vi "GET_OperatorsTable.vi"(8 "error in (no error)":errorcluster, 11 "Database Ref In":T1) -> (0 "error out":errorcluster, 2 "Array":string[][](array[string]), 3 "Database Ref Out":T1)   [LabVIEW 2018, in "MySQLTools.lvlib"]
uses:
  MySQLTools.lvlib
  <vilib>/addons/database/Connection.llb/Conn ObjectReference.ctl
  TypeDefs/DatabaseState.ctl
  <vilib>/addons/database/Recordset.llb/Rec ObjectReference.ctl
  <vilib>/addons/database/Auxilliary.llb/DB Tools Cursor Type.ctl
  <vilib>/addons/database/Connection.llb/Conn Execute.vi
  <vilib>/addons/database/Recordset.llb/Rec Fetch Recordset Data (R).vi
  <vilib>/addons/database/NI_Database_API.lvlib
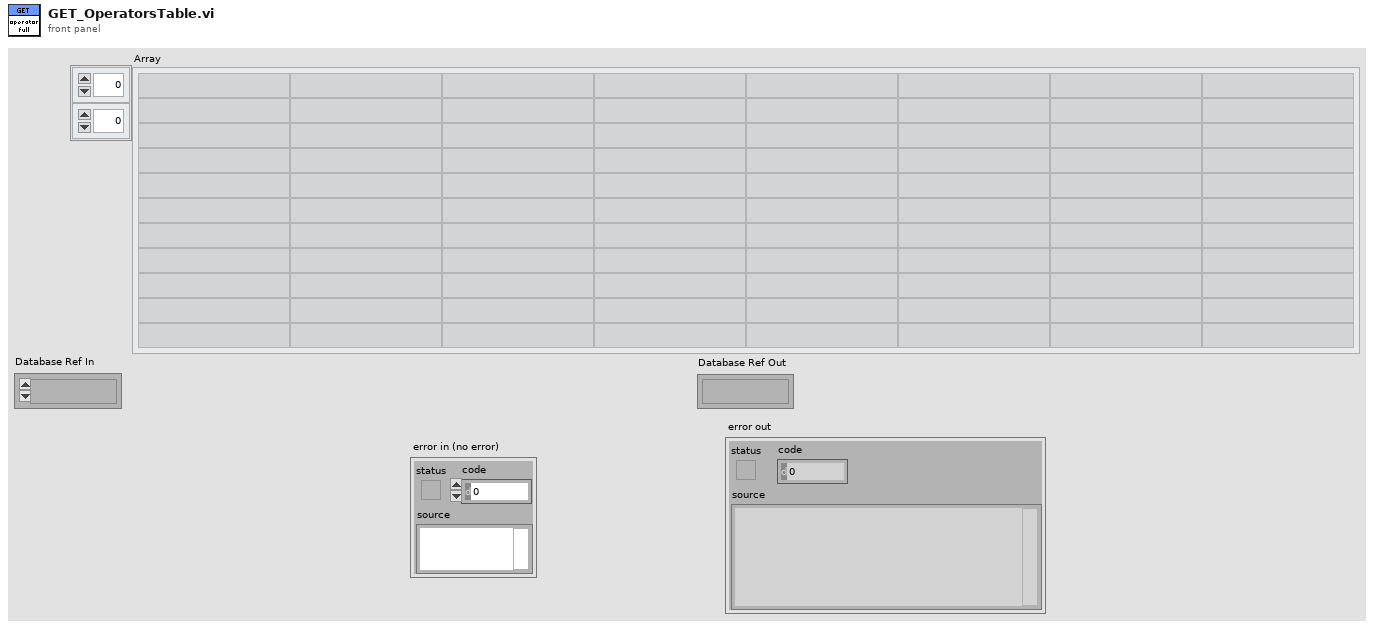
[diagram p1: front panel]
types:
  T1 = typedef "NI_Database_API.lvlib/Conn ObjectReference.ctl" = refnum<k1>
  T2 = typedef "NI_Database_API.lvlib/Rec ObjectReference.ctl" = refnum<k1>
  T3 = typedef "MySQLTools.lvlib/DatabaseState.ctl" = enum16{"Initialize", "Get Records", "Exit"}
  T4 = typedef "NI_Database_API.lvlib/DB Tools Cursor Type.ctl" = enum16{"forward-only", "keyset", "dynamic", "static"}
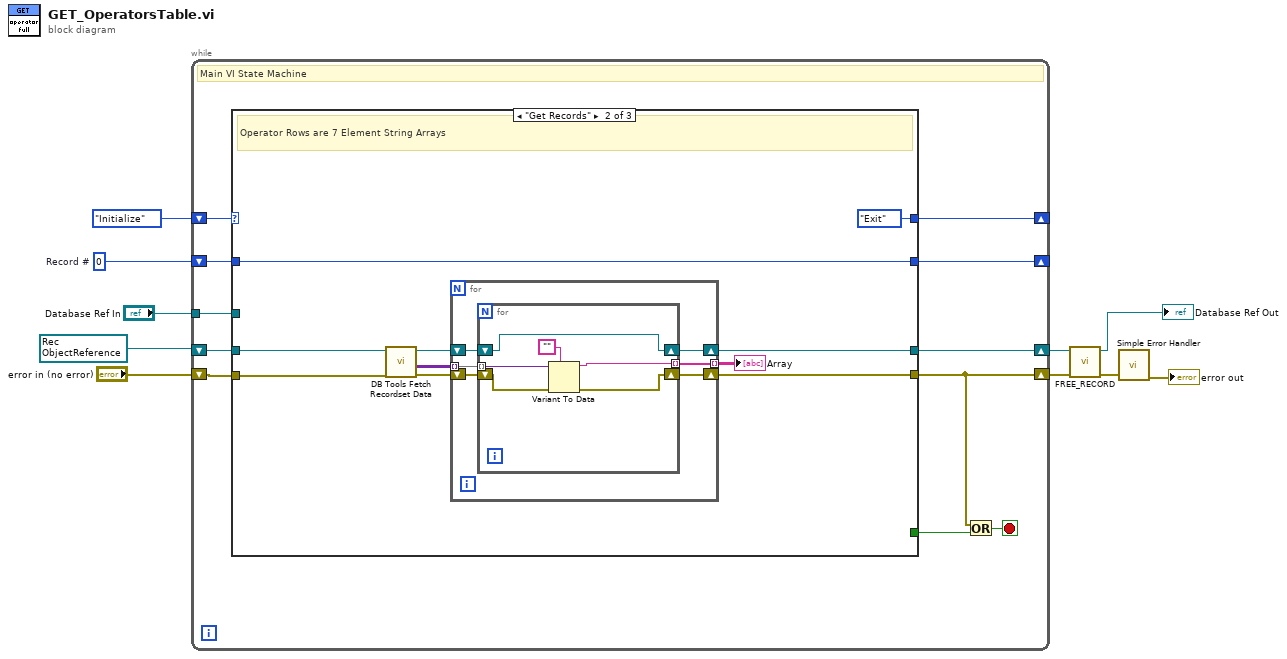
[diagram p0: block diagram]
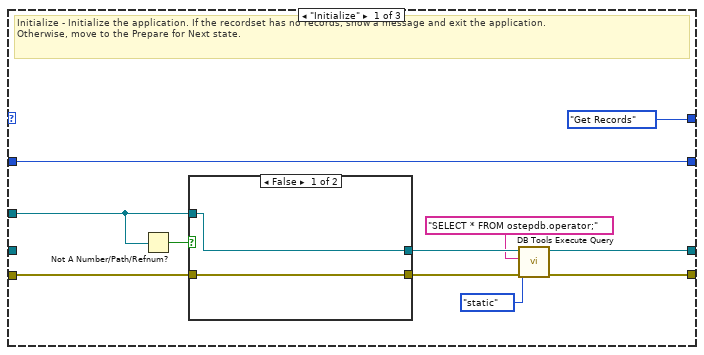
[diagram p2: hidden frame]
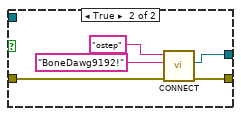
[diagram p3: hidden frame]
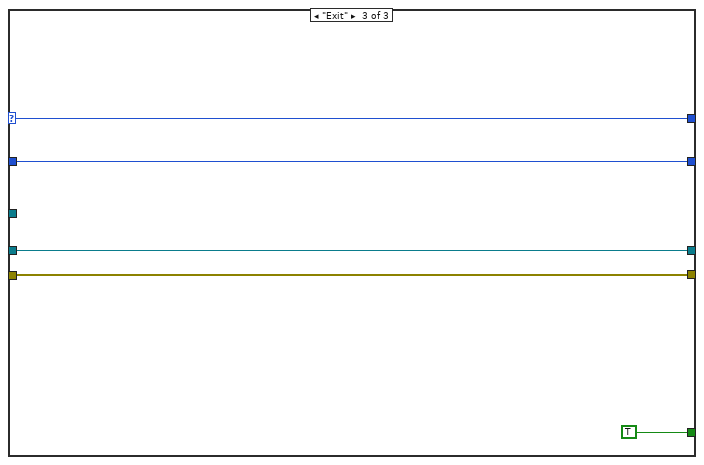
[diagram p4: hidden frame]
diagram:
  w2 = T2 refnum items=["Recordset"] ("recordset reference")
  w3 = u16 0  # Record #
  n1 = while {
    shift-right: [w17] -> w7
    shift-left: "error in (no error)" -> [w21]
    shift-right: [w20] -> _
    shift-left: DatabaseState."Initialize" ("State") -> [w19]
    shift-right: [w12] -> w4
    shift-left: w2 -> [w16]
    shift-right: [w14] -> _
    shift-left: w3 -> [w15]
    tunnel: "Database Ref In" -> [w11]
    stop <- w18 stop-if-true
    # "Main VI State Machine"
    n2 = case shown="\"Get Records\"" w19 {
      selector: w19 -> [_ _ w66]
      tunnel: w21 -> [w32 w47 w64]
      tunnel: [w28 w42 w64] -> w17
      tunnel: [DatabaseState."Get Records" ("State") DatabaseState."Exit" ("State") w66] -> w20
      tunnel: w16 -> [_ w48 w62]
      tunnel: w15 -> [w31 w49 w65]
      tunnel: [w31 w49 w65] -> w14
      tunnel: [_ _ TRUE] -> w13
      tunnel: [w26 w43 w62] -> w12
      tunnel: w11 -> [w22 _ _]
      frame "Initialize" {
        # "Initialize - Initialize the application. If the recordset has no records, show a message and exit the application. \nOtherwise, move to the Prepare for Next state."
        n3 = Not A Number/Path/Refnum?(number/path/refnum=w22) -> (NaN/Path/Refnum?=w23:bool)
        n4 = case shown="False" w23 {
          tunnel: w32 -> [w33 w39]
          tunnel: [w34 w35] -> w30
          tunnel: [w33 w38] -> w29
          tunnel: w22 -> [w34 _]
          frame False {
          }
          frame True {
            n5 = call "CONNECT.vi"("error in (no error)"=w39, "PASSWORD"="BoneDawg9192!" ("USER"), "USER"="ostep") -> ("error out"=w38:errorcluster, "connection ref out"=w35:T1)  [unwired: 7 in]
          }
        }
        n6 = call-poly <vilib>:"DB Tools Execute Query.vi"("error in (no error)"=w29, "cursor type"=DB_Tools_Cursor_Type."static", "SQL query"="SELECT * FROM ostepdb.operator;", "connection reference"=w30) -> ("error out"=w28:errorcluster, "recordset reference"=w26:T2)  [unwired: 4 in]
      }
      frame "Get Records" {
        # "Operator Rows are 7 Element String Arrays"
        n7 = call-poly <vilib>:"DB Tools Fetch Recordset Data.vi"("error in (no error)"=w47, "recordset reference"=w48) -> ("error out"=w45:errorcluster, "recordset data"=w44:variant[][], "recordset reference out"=w46:T2)  [unwired: 3 in]
        n8 = for {
          tunnel: w44 -> [w53] mode=indexing
          shift-right: [w52] -> w43
          shift-left: w46 -> [w55]
          shift-right: [w51] -> w42
          shift-left: w45 -> [w54]
          tunnel: [w50] -> w41 mode=indexing
          n9 = for {
            tunnel: w53 -> [w61] mode=indexing
            shift-right: [w57] -> w51
            shift-left: w54 -> [w60]
            shift-right: [w58] -> w52
            shift-left: w55 -> [w58]
            tunnel: [w56] -> w50 mode=indexing
            n10 = Variant To Data(error in=w60, type="", Variant=w61) -> (data=w56:string, error out=w57:errorcluster)
          }
        }
        "Array" <- w41
      }
      frame "Exit" {
      }
    }
    n11 = Or(x=w17, y=w13) -> (x .or. y?=w18:bool)
  }
  n12 = call "FREE_RECORD.vi"("error in (no error)"=w7, "Recordset Ref In"=w4) -> ("error out"=w6:errorcluster, "connection ref Out"=→"Database Ref Out":T1)  [unwired: 8 in]
  n13 = call <vilib>:"Simple Error Handler.vi"("error in (no error)"=w6) -> ("error out"=→"error out":errorcluster)  [unwired: 4 in, 4 out]
